vi "ShowConfigPage.vi"(8 "error in (no error)":errorcluster, 10 "Ancestor":string, 11 "Driver in":refnum<class "ViPER.lvclass">) -> (0 "error out":errorcluster, 3 "Driver out":refnum<class "ViPER.lvclass">)   [LabVIEW 2022 SP3, in "ViPER.lvlib" / "ViPER.lvclass"]
doc: "### BSD License (http://www.opensource.org/licenses/bsd-license.php) Begin ###\n\nCopyright (c) 2018 Kurt Friday www.medulla.net\n\nAll rights reserved.\n\nRedistribution and use in source and binary forms, with or without\nmodification, are permitted provided that the following conditions are met:\n\n * Redistributions of source code must retain the above copyright\n notice, this list of conditions and the following disclaimer.\n\n * Redistributions in binary form must reproduce the above copyright\n notice, this list of conditions and the following disclaimer in the\n documentation and/or other materials provided with the distribution.\n\n * Neither the name of the <organization> nor the\n names of its contributors may be used to endorse or promote products\n derived from this software without specific prior written permission.\n\nTHIS SOFTWARE IS PROVIDED BY THE COPYRIGHT HOLDERS AND CONTRIBUTORS \"AS IS\" AND\nANY EXPRESS OR IMPLIED WARRANTIES, INCLUDING, BUT NOT LIMITED TO, THE IMPLIED\nWARRANTIES OF MERCHANTABILITY AND FITNESS FOR A PARTICULAR PURPOSE ARE\nDISCLAIMED. IN NO EVENT SHALL <COPYRIGHT HOLDER> BE LIABLE FOR ANY\nDIRECT, INDIRECT, INCIDENTAL, SPECIAL, EXEMPLARY, OR CONSEQUENTIAL DAMAGES\n(INCLUDING, BUT NOT LIMITED TO, PROCUREMENT OF SUBSTITUTE GOODS OR SERVICES;\nLOSS OF USE, DATA, OR PROFITS; OR BUSINESS INTERRUPTION) HOWEVER CAUSED AND\nON ANY THEORY OF LIABILITY, WHETHER IN CONTRACT, STRICT LIABILITY, OR TORT\n(INCLUDING NEGLIGENCE OR OTHERWISE) ARISING IN ANY WAY OUT OF THE USE OF THIS\nSOFTWARE, EVEN IF ADVISED OF THE POSSIBILITY OF SUCH DAMAGE."
uses:
  ViPER.lvclass
panel:
  # "### BSD License (http://www.opensource.org/licenses/bsd-license.php) Begin ###\n\nCopyright (c) 2018  Kurt Friday www.medulla.net\n\nAll rights reserved.\n\nRedistribution and use in source and binary forms, with or without\nmodification, are permitted provided that the following conditions are met:\n\n    * Redistributions of source code must retain the above copyright\n      notice, this list of conditions and the following disclaimer.\n\n    * Redistributions in binary form must reproduce the above copyright\n      notice, this list of conditions and the following disclaimer in the\n      documentation and/or other materials provided with the distribution.\n\n    * Neither the name of the <organization> nor the\n      names of its contributors may be used to endorse or promote products\n      derived from this software without specific prior written permission.\n\nTHIS SOFTWARE IS PROVIDED BY THE COPYRIGHT HOLDERS AND CONTRIBUTORS \"AS IS\" AND\nANY EXPRESS OR IMPLIED WARRANTIES, INCLUDING, BUT NOT LIMITED TO, THE IMPLIED\nWARRANTIES OF MERCHANTABILITY AND FITNESS FOR A PARTICULAR PURPOSE ARE\nDISCLAIMED. IN NO EVENT SHALL <COPYRIGHT HOLDER> BE LIABLE FOR ANY\nDIRECT, INDIRECT, INCIDENTAL, SPECIAL, EXEMPLARY, OR CONSEQUENTIAL DAMAGES\n(INCLUDING, BUT NOT LIMITED TO, PROCUREMENT OF SUBSTITUTE GOODS OR SERVICES;\nLOSS OF USE, DATA, OR PROFITS; OR BUSINESS INTERRUPTION) HOWEVER CAUSED AND\nON ANY THEORY OF LIABILITY, WHETHER IN CONTRACT, STRICT LIABILITY, OR TORT\n(INCLUDING NEGLIGENCE OR OTHERWISE) ARISING IN ANY WAY OUT OF THE USE OF THIS\nSOFTWARE, EVEN IF ADVISED OF THE POSSIBILITY OF SUCH DAMAGE."
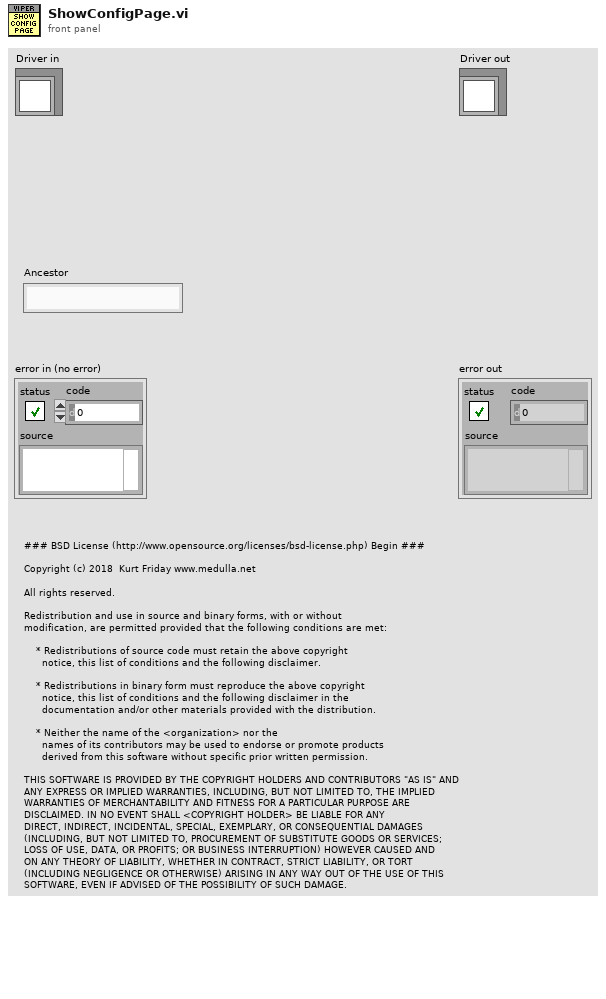
[diagram p1: front panel]
types:
  T1 = typedef "ViPER.lvlib/ViPER.lvclass/Details.ctl" = cluster{"Name":string, "Class":string}
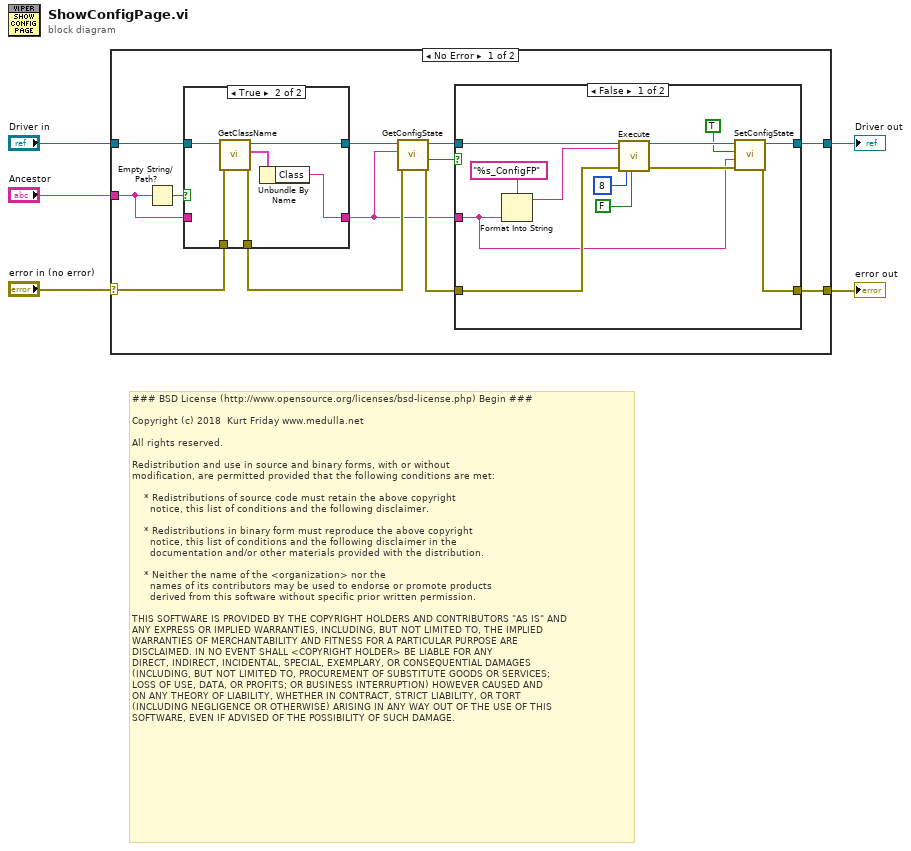
[diagram p0: block diagram]
diagram:
  # "### BSD License (http://www.opensource.org/licenses/bsd-license.php) Begin ###\n\nCopyright (c) 2018  Kurt Friday www.medulla.net\n\nAll rights reserved.\n\nRedistribution and use in source and binary forms, with or without\nmodification, are permitted provided that the following conditions are met:\n\n    * Redistributions of source code must retain the above copyright\n      notice, this list of conditions and the following disclaimer.\n\n    * Redistributions in binary form must reproduce the above copyright\n      notice, this list of conditions and the following disclaimer in the\n      documentation and/or other materials provided with the distribution.\n\n    * Neither the name of the <organization> nor the\n      names of its contributors may be used to endorse or promote products\n      derived from this software without specific prior written permission.\n\nTHIS SOFTWARE IS PROVIDED BY THE COPYRIGHT HOLDERS AND CONTRIBUTORS \"AS IS\" AND\nANY EXPRESS OR IMPLIED WARRANTIES, INCLUDING, BUT NOT LIMITED TO, THE IMPLIED\nWARRANTIES OF MERCHANTABILITY AND FITNESS FOR A PARTICULAR PURPOSE ARE\nDISCLAIMED. IN NO EVENT SHALL <COPYRIGHT HOLDER> BE LIABLE FOR ANY\nDIRECT, INDIRECT, INCIDENTAL, SPECIAL, EXEMPLARY, OR CONSEQUENTIAL DAMAGES\n(INCLUDING, BUT NOT LIMITED TO, PROCUREMENT OF SUBSTITUTE GOODS OR SERVICES;\nLOSS OF USE, DATA, OR PROFITS; OR BUSINESS INTERRUPTION) HOWEVER CAUSED AND\nON ANY THEORY OF LIABILITY, WHETHER IN CONTRACT, STRICT LIABILITY, OR TORT\n(INCLUDING NEGLIGENCE OR OTHERWISE) ARISING IN ANY WAY OUT OF THE USE OF THIS\nSOFTWARE, EVEN IF ADVISED OF THE POSSIBILITY OF SUCH DAMAGE."
  n1 = case shown="No Error" "error in (no error)" {
    selector: "error in (no error)" -> [w12 w42]
    tunnel: [w16 w42] -> w4
    tunnel: [w17 w41] -> w2
    tunnel: "Driver in" -> [w10 w41]
    tunnel: "Ancestor" -> [w7 _]
    frame No Error {
      n2 = Empty String/Path?(string/path=w7) -> (empty?=w8:bool)
      n3 = case shown="True" w8 {
        tunnel: w12 -> [w19 w26]
        tunnel: [w19 w25] -> w11
        tunnel: w10 -> [w20 w24]
        tunnel: [w20 w23] -> w9
        tunnel: w7 -> [w18 _]
        tunnel: [w18 w21] -> w6
        frame False {
        }
        frame True {
          n4 = call "GetClassName.vi"("error in (no error)"=w26, "reference in"=w24) -> ("error out"=w25:errorcluster, "Details"=w22:T1, "reference out"=w23:refnum<class "ViPER.lvclass">)  [unwired: 7 in]
          n5 = Unbundle By Name(w22) -> ("Class"=w21:string)
        }
      }
      n6 = call-dynamic "GetConfigState.vi"("error in (no error)"=w11, "Ancestor"=w6, "reference in"=w9) -> ("error out"=w15:errorcluster, "config_open"=w14:bool, "reference out"=w13:refnum<class "ViPER.lvclass">)  [unwired: 6 in]
      n7 = case shown="False" w14 {
        tunnel: w15 -> [w38 w39]
        tunnel: w13 -> [w37 w40]
        tunnel: [w31 w39] -> w16
        tunnel: [w33 w40] -> w17
        tunnel: w6 -> [w27 _]
        frame False {
          n8 = Format Into String(format string="%s_ConfigFP" ("method"), w27) -> (resulting string=w28:string)  [unwired: 2 in, 1 out]
          n9 = call-dynamic "Execute.vi"("reference in"=w37, "cmd"=w28, "error in (no error)"=w38, "options"=8, "wait until done (T)"=FALSE) -> ("reference out"=w34:refnum<class "ViPER.lvclass">, "error out"=w32:errorcluster)  [unwired: 10 in, 3 out]
          n10 = call "SetConfigState.vi"("error in (no error)"=w32, "Ancestor"=w27, "Config Open"=TRUE, "reference in"=w34) -> ("error out"=w31:errorcluster, "reference out"=w33:refnum<class "ViPER.lvclass">)  [unwired: 6 in]
        }
        frame True {
        }
      }
    }
    frame Error {
    }
  }
  "error out" <- w4
  "Driver out" <- w2
